vi "calc.vi"(8 "y":dbl, 9 "r":dbl, 11 "Qube":refnum<class "Qube.lvclass">) -> (1 "u":dbl, 3 "Qube":refnum<class "Qube.lvclass">)   [LabVIEW 2017, in "Qube.lvclass"]
uses:
  Qube.lvclass
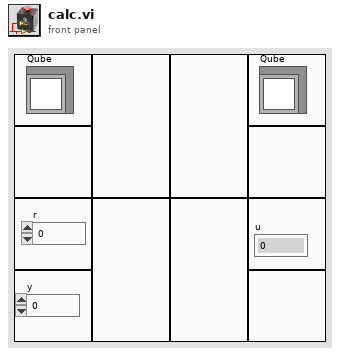
[diagram p1: front panel]
types:
  T1 = typedef "Qube.lvclass/mode.ctl" = enum16{"Control", "Identify"}
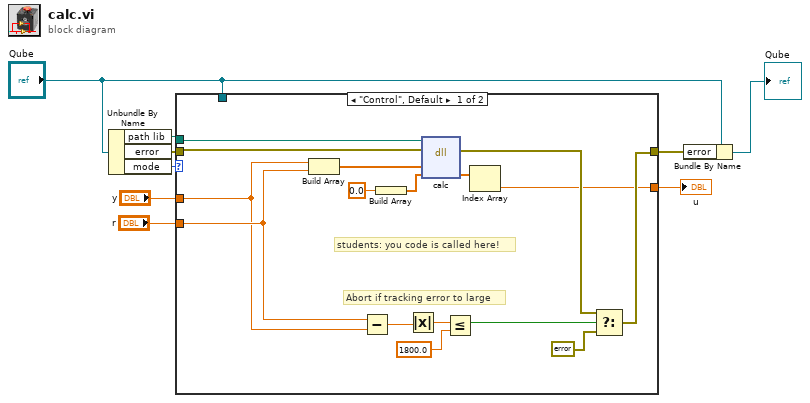
[diagram p0: block diagram]
diagram:
  n1 = Unbundle By Name("Qube") -> ("path lib"=w2:path, "error"=w1:errorcluster, "mode"=w5:T1)
  n2 = case shown="\"Control\", Default" w5 {
    tunnel: "Qube" -> [_ _]
    tunnel: [w15 w26] -> w8
    tunnel: [w14 w27] -> w7
    tunnel: "r" -> [w11 w27]
    tunnel: "y" -> [w10 _]
    tunnel: w2 -> [w13 _]
    tunnel: w1 -> [w12 w26]
    frame "Control", Default {
      # "students: you code is called here!"
      # "Abort if tracking error to large"
      n3 = Build Array(w10, w11) -> (w22:dbl[])
      n4 = Subtract(x=w11, y=w10) -> (x-y=w21:dbl)
      n5 = Build Array(0.0 ("element")) -> (w25:dbl[])
      n6 = Absolute Value(x=w21) -> (abs(x)=w20:dbl)
      n7 = dll-call lib="?" fn="calc"(path in=w13, error in=w12, "in"=w22, "out"=w25) -> (error out=w17:errorcluster, "out"=w23:dbl[])  [unwired: 3 in, 1 out]
      n8 = Less Or Equal?(x=w20, y=1800.0) -> (x <= y?=w18:bool)
      n9 = Index Array(array=w23) -> (element=w14:dbl)  [unwired: 1 in]
      n10 = Select(t=w17, s=w18, f=errorcluster {"status"=TRUE, "code"=1000, "source"="Tracking error to large"}) -> (s? t:f=w15:errorcluster)
    }
    frame "Identify" {
    }
  }
  "u" <- w7
  n11 = Bundle By Name(cluster="Qube", "error"=w8) -> (→"Qube":refnum<class "Qube.lvclass">)
